vi "Set Auto Config Dev Lv.vi"(8 "error in (no error)":errorcluster, 10 "fAutoConfig":i32, 11 "hdwf":i32) -> (0 "error out":errorcluster, 1 "function return":i32, 3 "hdwf out":i32)   [LabVIEW 2013, in "AnalogDiscSDKLv.lvlib"]
doc: "extern \"C\" __declspec(dllexport) int SetAutoConfig_DevLv(HDWF hdwf, int fAutoConfig);"
uses:
  <instrlib>/AnalogDiscSDKLv/AnalogDiscSDKLv.lvlib
  <instrlib>/AnalogDiscSDKLv/AnalogDiscSDKLv.dll
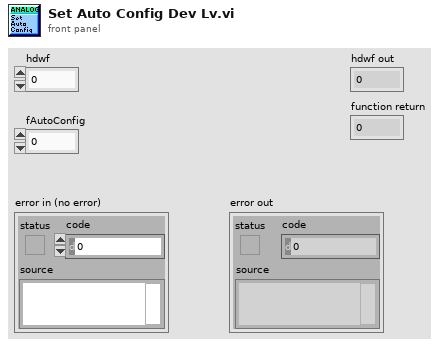
[diagram p1: front panel]
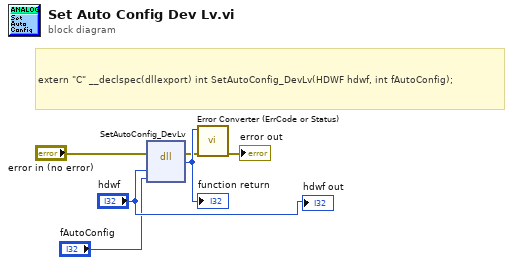
[diagram p0: block diagram]
diagram:
  # "extern \"C\" __declspec(dllexport) int SetAutoConfig_DevLv(HDWF hdwf, int fAutoConfig);"
  n1 = dll-call lib="C:/Program Files (x86)/National Instruments/LabVIEW 2013/instr.lib/AnalogDiscSDKLv/AnalogDiscSDKLv.*" fn="SetAutoConfig_DevLv"(error in="error in (no error)", "hdwf"="hdwf", "fAutoConfig"="fAutoConfig") -> (error out=w2:errorcluster, w6:i32)  [unwired: 4 in, 1 out]
  "function return" <- w6
  n2 = call <instrlib>:"Error Converter (ErrCode or Status).vi"("error in (no error)"=w2, "error code"=w6) -> ("error out"=→"error out":errorcluster)  [unwired: 9 in]
  "hdwf out" <- "hdwf"
